vi "FGA Get Waypoint Count.vi"() -> (0 "count":u16)   [LabVIEW 2009]
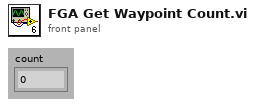
[diagram p1: front panel]
types:
  T1 = typedef "RequestIDRec.ctl" = cluster{"RequestId":u8, "Element List":T2[]}
  T2 = typedef "ElementRec.ctl" = cluster{"ElementUID":u16, " PreviousUID":u16, " NextUID":u16, "LocalWaypointRec":T3}
  T3 = typedef "LocalWaypointRec.ctl" = cluster{"Presence Vector":u8, " X":dbl, " Y":dbl, " Z":dbl, "Roll":dbl, "Pitch":dbl, "Yaw":dbl, "Waypoint Tolerance":dbl, "Path Tolerance":dbl, "Is Active?":bool}
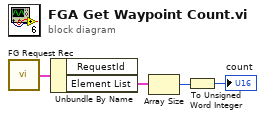
[diagram p0: block diagram]
diagram:
  n1 = call "FG Request Rec.vi"() -> ("Request out"=w4:T1)  [unwired: 2 in]
  n2 = Unbundle By Name(w4) -> ("Element List"=w3:T2[])  [unwired: 1 out]
  n3 = Array Size(array=w3) -> (size(s)=w1:i32)
  n4 = To Unsigned Word Integer(number=w1) -> (unsigned 16bit integer=→"count":u16)
